vi "Copy of Find_tuned_T1_T2.vi"(9 "Tmaster to":dbl=30.0, 10 "Tslave from":dbl=79.025, 11 "Tmaster from":dbl=75.0) -> (1 "dTslave":dbl=-31.964547910252442 format="%.2g", 2 "dT1":dbl=-45.0, 3 "Tslave  to":dbl=47.060452089747564)   [LabVIEW 2010]
panel:
  out "Order 2":dbl=210.0 format="%.1f"
  out "Order 1":dbl=210.0 format="%.1f"
  out "Dt 2":dbl[](array[numeric])=[-49.0289488656166, -31.436555634993937, -24.131748637488926, -20.93789708119516] format="%.1f"
  out "Dt 1":dbl[](array[numeric])=[-45.0029581682178, -37.906138342994396, -27.913435789189037, -23.77116322813478] format="%.1f"
  out "Temperature orders Et1 2":dbl[](array[numeric])=[30.0, 79.0289488656166, 110.46550450061054, 134.59725313809946, 155.53515021929462] format="%.1f"
  out "Temperature orders Et1":dbl[](array[numeric])=[30.0, 75.0029581682178, 112.9090965112122, 140.82253230040124, 164.59369552853602] format="%.1f"
  in  "Wavelength":dbl=1.28 format="%_6g"
  in  "Et slave thickness":dbl=250.0 format="%.1f"
  in  "Etmaster  thickness":dbl=210.0 format="%.1f"
  out "Tslave @ vortex":dbl=30.0 format="%.2g"
  out "Out of  Range":bool
  out "Tmaster @ vortex":dbl=30.0 format="%.2g"
  in  "Angle from":dbl=8.0
  out "dV":dbl=361.67430149747213
  out "Angle TO":dbl=9.893115982240609
  out "dTslave/dTmaster":dbl=0.7103232868944988
  out "refr inx slave  to":dbl=3.511376728547932
  out "refr inx slave from":dbl=3.5128179592813007
  out "refr inx master to":dbl=3.51113
  out "refr inx master from":dbl=3.512571129464609
  out "Temperature vs refractive index":cluster{"Refr index raw":dbl[], "yi":dbl[]}[](graph)=[{"Refr index raw"=[3.51113, 3.51123, 3.51146, 3.51181, 3.51229, 3.51288, 3.51358, 3.51439, 3.51979, 3.52703, 3.53555, 3.54394], "yi"=[30.0, 40.0, 50.0, 60.0, 70.0, 80.0, 90.0, 100.0, 150.0, 200.0, 250.0, 295.0]}, {"Refr index raw"=[3.511376728547932], "yi"=[47.060452089747564]}]
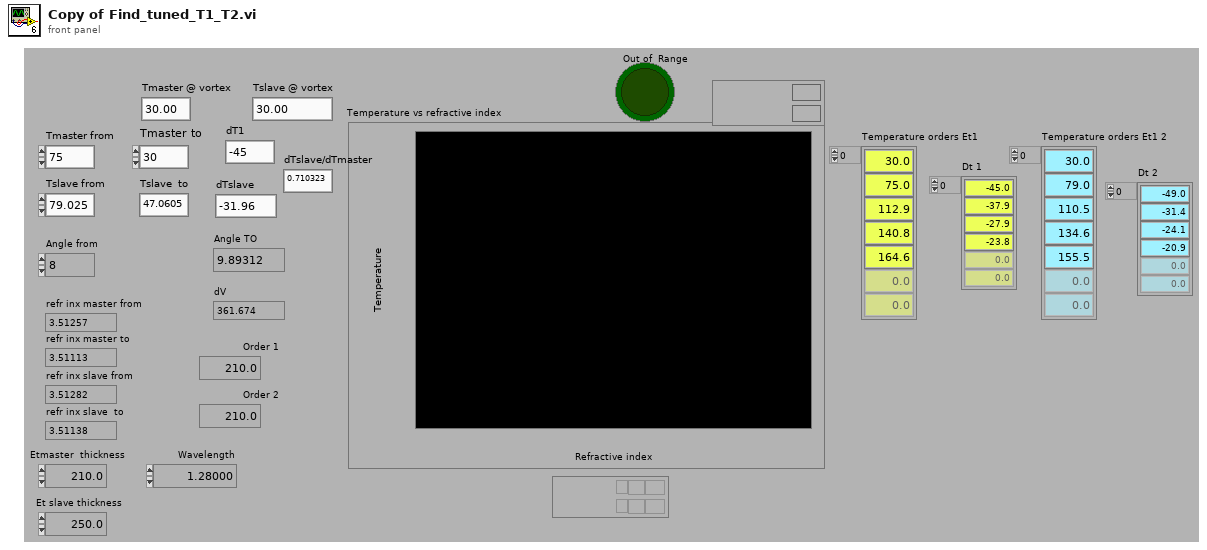
[diagram p1: front panel]
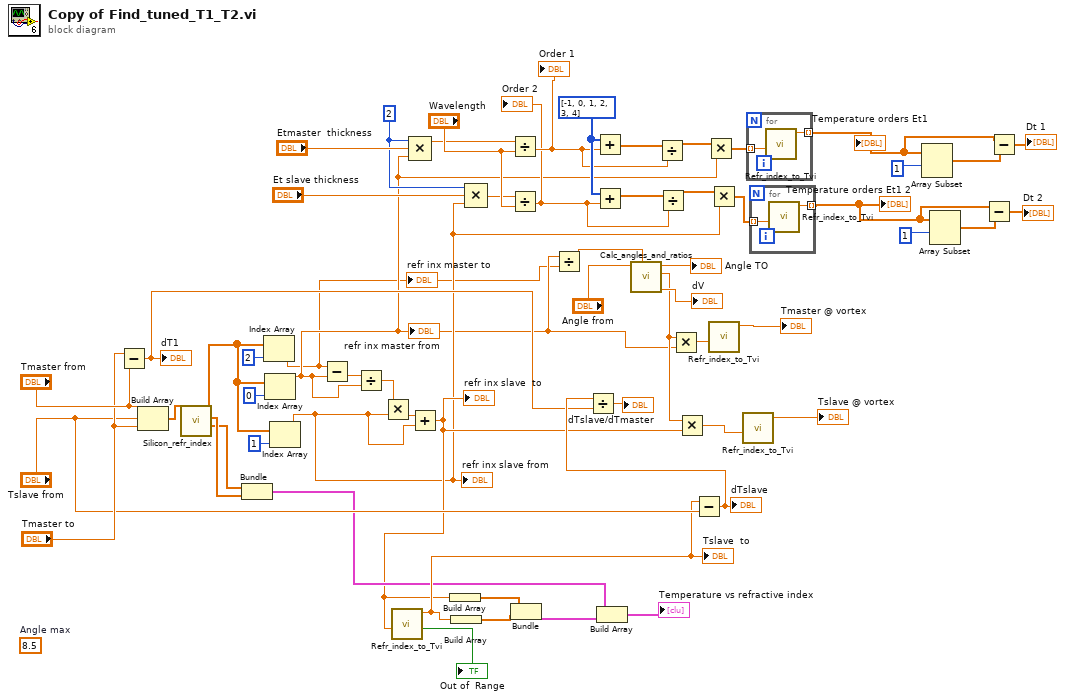
[diagram p0: block diagram]
diagram:
  w13 = 2 ("index")
  w23 = i32[] [-1, 0, 1, 2, 3, 4]
  (unwired) 8.5  # Angle max
  n1 = Subtract(x="Tmaster to", y="Tmaster from") -> (x-y=w46:dbl)
  "dT1" <- w46
  n2 = Build Array("Tmaster from", "Tslave from", "Tmaster to") -> (w58:dbl[])
  n3 = call "Silicon_refr_index.vi"("Temperature"=w58) -> ("Refr index raw"=w40:dbl[], "T raw"=w41:dbl[], "Silicon refr index at T"=w53:dbl[])  [unwired: 8 in]
  n4 = Bundle("Refr index raw"=w40, "T raw"=w41) -> (w39:cluster{"Refr index raw":dbl[], "T raw":dbl[]})  [unwired: 1 in]
  n5 = Index Array(array=w53, index=2) -> (element=w1:dbl)
  "refr inx master to" <- w1
  n6 = Index Array(array=w53, index=0) -> (element=w2:dbl)
  "refr inx master from" <- w2
  n7 = Index Array(array=w53, index=1) -> (element=w17:dbl)
  "refr inx slave from" <- w17
  n8 = Subtract(x=w1, y=w2) -> (x-y=w54:dbl)
  n9 = Divide(x=w54, y=w2) -> (x/y=w52:dbl)
  n10 = Multiply(x=w52, y=w17) -> (x*y=w51:dbl)
  n11 = Compound Arithmetic op=MULTIPLY(w13, "Etmaster  thickness", w2) -> (w21:dbl)
  n12 = Add(x=w51, y=w17) -> (x+y=w28:dbl)
  "refr inx slave  to" <- w28
  n13 = call "Refr_index_to_Tvi.vi"("refr inx"=w28) -> ("Out of  Range"=→"Out of  Range":bool, "T tune to"=w42:dbl)  [unwired: 9 in]
  "Tslave  to" <- w42
  n14 = Build Array(w28) -> (w44:dbl[])
  n15 = Build Array(w42) -> (w43:dbl[])
  n16 = Compound Arithmetic op=MULTIPLY(w13, "Et slave thickness", w17) -> (w14:dbl)
  n17 = Divide(x=w21, y="Wavelength") -> (x/y=w4:dbl)
  "Order 1" <- w4
  n18 = Divide(x=w14, y="Wavelength") -> (x/y=w3:dbl)
  "Order 2" <- w3
  n19 = Bundle(w44, w43) -> (w38:cluster{dbl[], dbl[]})  [unwired: 1 in]
  n20 = Divide(x=w2, y=w1) -> (x/y=w35:dbl)
  n21 = Add(x=w23, y=w4) -> (x+y=w22:dbl[])
  n22 = Add(x=w23, y=w3) -> (x+y=w20:dbl[])
  n23 = Build Array(w39, w38) -> (→"Temperature vs refractive index":cluster{"Refr index raw":dbl[], "T raw":dbl[]}[])
  n24 = call "Calc_angles_and_ratios.vi"("COS ratio (TO/FROM) - internal"=w35, "Angle FROM deg (ext)"="Angle from") -> ("V at angle TO"=→"dV":dbl, "Cos  FROM  (internal)"=w27:dbl, "Angle TO  deg (ext)"=→"Angle TO":dbl)  [unwired: 6 in, 1 out]
  n25 = Divide(x=w22, y=w4) -> (x/y=w19:dbl[])
  n26 = Divide(x=w20, y=w3) -> (x/y=w18:dbl[])
  n27 = Multiply(x=w27, y=w2) -> (x*y=w32:dbl)
  n28 = Multiply(x=w27, y=w28) -> (x*y=w30:dbl)
  n29 = Subtract(x=w42, y="Tslave from") -> (x-y=w47:dbl)
  "dTslave" <- w47
  n30 = Divide(x=w47, y=w46) -> (x/y=→"dTslave/dTmaster":dbl)
  n31 = Multiply(x=w19, y=w2) -> (x*y=w16:dbl[])
  n32 = Multiply(x=w18, y=w17) -> (x*y=w15:dbl[])
  n33 = call "Refr_index_to_Tvi.vi"("refr inx"=w32) -> ("T tune to"=→"Tmaster @ vortex":dbl)  [unwired: 9 in, 1 out]
  n34 = call "Refr_index_to_Tvi.vi"("refr inx"=w30) -> ("T tune to"=→"Tslave @ vortex":dbl)  [unwired: 9 in, 1 out]
  n35 = for {
    tunnel: w16 -> [w61] mode=indexing
    tunnel: [w60] -> w11 mode=indexing
    n36 = call "Refr_index_to_Tvi.vi"("refr inx"=w61) -> ("T tune to"=w60:dbl)  [unwired: 9 in, 1 out]
  }
  "Temperature orders Et1" <- w11
  n37 = for {
    tunnel: w15 -> [w63] mode=indexing
    tunnel: [w62] -> w8 mode=indexing
    n38 = call "Refr_index_to_Tvi.vi"("refr inx"=w63) -> ("T tune to"=w62:dbl)  [unwired: 9 in, 1 out]
  }
  "Temperature orders Et1 2" <- w8
  n39 = Array Subset(array=w11, index=1) -> (w10:dbl[])  [unwired: 1 in]
  n40 = Array Subset(array=w8, index=1) -> (w7:dbl[])  [unwired: 1 in]
  n41 = Subtract(x=w8, y=w7) -> (x-y=→"Dt 2":dbl[])
  n42 = Subtract(x=w11, y=w10) -> (x-y=→"Dt 1":dbl[])
